vi "Fill.vi"(4 "Use New Fill Algorithm? (F)":bool, 5 "Tool filling? (T)":bool=TRUE, 6 "Ref Color":u32(colorbox)=16777215, 7 "rect":T1={"left"=0, "top"=0, "right"=32, "bottom"=32}, 9 "Pic Mouse Down":T2={"Horizontal"=16, "Vertical"=17}, 10 "New Color":u32(colorbox)=16777214, 11 "Pic In":picture) -> (3 "Pic Out":picture)   [LabVIEW 2020, in "lv_icon.lvlib"]
doc: "Run the Fill Algorithm."
uses:
  resource/plugins/lv_icon.lvlib
  <vilib>/Utility/miscctls.llb/LVPoint32TypeDef.ctl
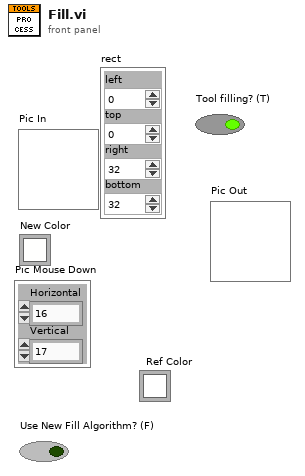
[diagram p1: front panel]
types:
  T1 = cluster{"left":i16, "top":i16, "right":i16, "bottom":i16}
  T2 = typedef "LVPoint32TypeDef.ctl" = cluster{"Horizontal":i32, "Vertical":i32}
  T3 = typedef "imagedata.ctl" = cluster{"image type":i32, "image depth":i32, "image":u8[], "mask":u8[], "colors":u32[], "Rectangle":cluster{"left":i16, "top":i16, "right":i16, "bottom":i16}}
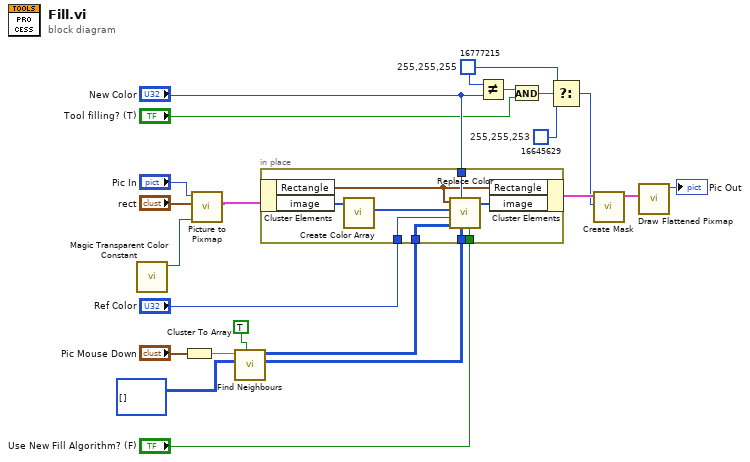
[diagram p0: block diagram]
diagram:
  w4 = u32 16645629  # 255,255,253
  w5 = u32 16777215  # 255,255,255
  n1 = call "Magic Transparent Color Constant.vi"() -> ("Magic transparent color constant"=w8:u32)  [unwired: 11 out]
  n2 = Cluster To Array(cluster="Pic Mouse Down") -> (array=w21:i32[])
  n3 = call <vilib>:"Picture to Pixmap.vi"("Background Color"=w8, "rect"="rect", "picture"="Pic In") -> ("image data"=w13:T3)  [unwired: 1 in, 7 out]
  n4 = call "Find Neighbours.vi"("Add Start Point?"=TRUE, "Points In"=i32[][] [], "XY"=w21) -> ("Points out"=w11:i32[][], "Filtered"=w20:i32[][])  [unwired: 1 in, 6 out]
  n5 = in-place {
    in-place-border: w20 -> [w31]
    in-place-border: "New Color" -> [w29]
    in-place-border: "Ref Color" -> [w28]
    in-place-border: w11 -> [w25]
    in-place-border: "Use New Fill Algorithm? (F)" -> [w23]
    n6 = in-place-cluster #1(w13) -> ("Rectangle"=w24:T1, "image"=w27:u8[])
    n7 = call "Create Color Array.vi"("RGB in"=w27) -> ("U32 color"=w26:u32[])  [unwired: 10 out]
    n8 = call "Replace Color.vi"("Use New Fill Algorithm? (F)"=w23, "Points In"=w25, "New Color"=w29, "5 Pixels"=w31, "Ref Color"=w28, "U32 color"=w26, "Rectangle"=w24) -> ("RGB out"=w30:u8[])  [unwired: 1 in, 3 out]
    n9 = in-place-cluster #1("Rectangle"=w24, "image"=w30) -> (w19:T3)
  }
  n10 = Not Equal?(x=w5, y="New Color") -> (x != y?=w3:bool)
  n11 = And(x=w3, y="Tool filling? (T)") -> (x .and. y?=w2:bool)
  n12 = Select(t=w5, s=w2, f=w4) -> (s? t:f=w6:u32)
  n13 = call <vilib>:"Create Mask.vi"("Mask Color (Black)"=w6, "image data"=w19) -> ("image data"=w18:T3)  [unwired: 2 in, 7 out]
  n14 = call <vilib>:"Draw Flattened Pixmap.vi"("image data"=w18) -> ("new picture"=→"Pic Out":picture)  [unwired: 1 in, 7 out]
